vi "Autonomous Independent.vi"() -> ()   [LabVIEW 2015]
doc: "This VI is called when autonomous begins, and will automatically be terminated when autonomous ends. You can carry out timed or sensor driven robot movement independently without needing to return to the caller."
uses:
  navX-MXP Library/COMMON/TypeDefs/Data TypeDefs/navX Vector Data.ctl
  navX-MXP Library/COMMON/TypeDefs/Data TypeDefs/navX YPRH Data.ctl
  navX-MXP Library/COMMON/TypeDefs/Data TypeDefs/navX Quaternion Data.ctl
  Robot Global Data.vi
  navX-MXP Library/navX-MXP IMU.lvlib
  <vilib>/addons/control/pid/NI_PID_pid.lvlib
  <vilib>/addons/control/pid/pid.llb/PID (DBL).vi
panel:
  in  "PID gains":T1={"proportional gain (Kc)"=1.0, "integral time (Ti, min)"=0.01, "derivative time (Td, min)"=0.0} {"derivative time (Td, min)" format="%.3f"; "integral time (Ti, min)" format="%.3f"; "proportional gain (Kc)" format="%.3f"}
  in  "Drive Speed":dbl
  out "Quaternion":T2
  out "YPRH":T3
  out "Raw Magnetometer":T4
  out "Raw Gyro":T4
  out "Raw Acceleration":T4
  out "Fused Heading":dbl
  # "Be sure to right-click and choose Data Operations>>Make Current Value default if you want to save the array values with the VI"
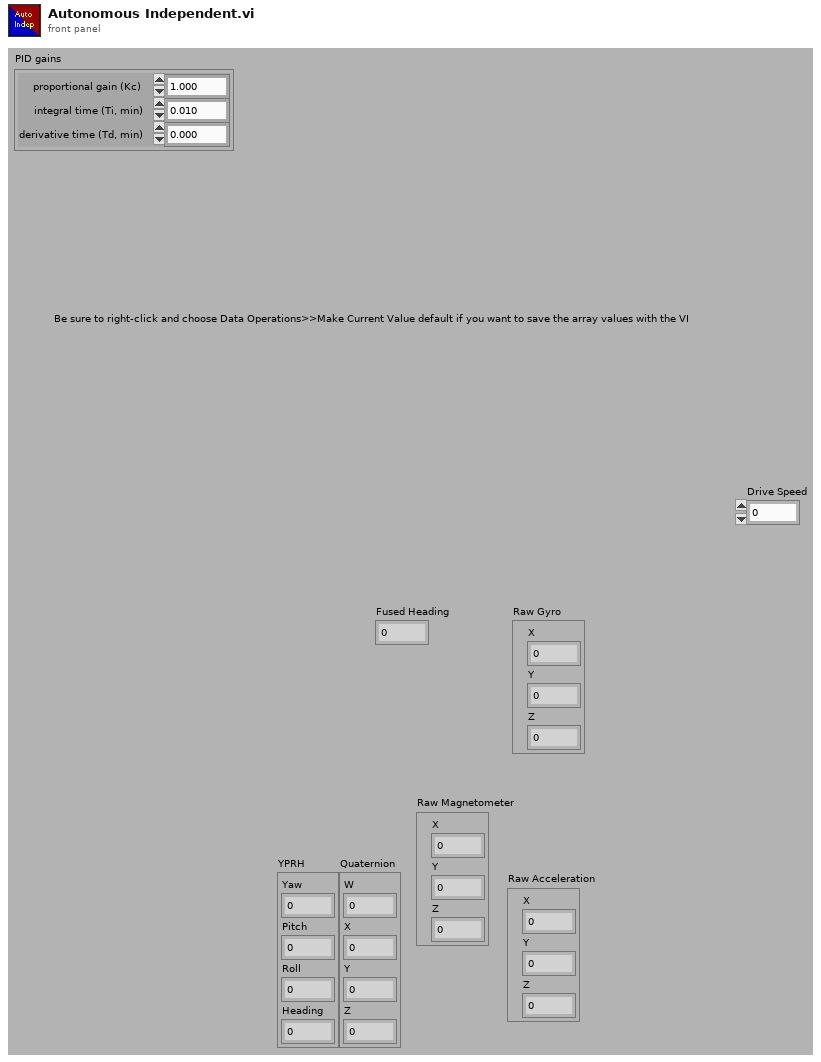
[diagram p1: front panel]
types:
  T1 = cluster{"proportional gain (Kc)":dbl, "integral time (Ti, min)":dbl, "derivative time (Td, min)":dbl}
  T2 = typedef "navX-MXP IMU.lvlib/navX Quaternion Data.ctl" = cluster{"W":dbl, "X":dbl, "Y":dbl, "Z":dbl}
  T3 = typedef "navX-MXP IMU.lvlib/navX YPRH Data.ctl" = cluster{"Yaw":dbl, "Pitch":dbl, "Roll":dbl, "Heading":dbl}
  T4 = typedef "navX-MXP IMU.lvlib/navX Vector Data.ctl" = cluster{"X":dbl, "Y":dbl, "Z":dbl}
  T5 = typedef "navX-MXP IMU.lvlib/navX Device TypeDef.ctl" = cluster{"navX Interface Protocol":T6, "navX Interface Protocol TypeDefs":cluster{"SPIDevRef":T7, "I2CDevRef":T9}, "navX System Information":cluster{"Board Information":T11, "Status":T14, "Offsets":T18, "LastSampleTimestamp":dbl, "LastSampleValid":bool}, "navX Common Information":cluster{"Update Rate (4Hz-60Hz)":T19, "refnum name":string, "error":errorcluster, "LastSampleFPGATimestamp":dbl}}
  T6 = typedef "navX-MXP IMU.lvlib/navX Interface Protocol.ctl" = enum16{"SPI", "I2C", "SERIAL"}
  T7 = typedef "WPI_SPIDevRef.ctl" = cluster{"DevStatus":errorcluster, "Handle":i32, "SPI Bus":T8}
  T8 = typedef "spi_bus.ctl" = enum16{"SPI On-Board, CS0", "SPI On-Board, CS1", "SPI On-Board, CS2", "SPI On-Board, CS3", "SPI MXP", "Invalid"}
  T9 = typedef "WPI_I2CDevRef.ctl" = cluster{"DevStatus":errorcluster, "Device Address":u8, "Handle":i32, "I2C Bus":T10}
  T10 = typedef "i2c_bus.ctl" = enum16{"I2C On-Board", "I2C MXP", "Invalid"}
  T11 = typedef "navX-MXP IMU.lvlib/navX Board Information.ctl" = cluster{"WhoAmI (50 | 0x32)":u8, "Board Revision":u8, "Firmware Major Version":u8, "Firmware Minor Version":u8, "NAVX_BOARD_CAPABILITY":T12, "NAVX_BOARD_YAW_AXIS":T13}
  T12 = typedef "navX-MXP IMU.lvlib/navX NAVX_BOARD_CAPABILITY.ctl" = cluster{"OMNIMOUNT":bool, "YAW_RESET":bool, "VEL_AND_DISP":bool}
  T13 = typedef "navX-MXP IMU.lvlib/navX NAVX_BOARD_YAW_AXIS.ctl" = cluster{"BOARD_YAW_AXIS_UP":bool, "BOARD_YAW_AXIS":u8}
  T14 = typedef "navX-MXP IMU.lvlib/navX Status Data.ctl" = cluster{"Update Rate Hz":u8, "Accelerometer Full-Scale Range":u8, "Gyro Full-Scale Range":u16, "NAVX_OP_STATUS":T15, "NAVX_CAL_STATUS":T16, "NAVX_SELFTEST_STATUS":u8, "NAVX_SENSOR_STATUS":T17}
  T15 = typedef "navX-MXP IMU.lvlib/navX NAVX_OP_STATUS.ctl" = u8
  T16 = typedef "navX-MXP IMU.lvlib/navX NAVX_CAL_STATUS.ctl" = u8
  T17 = typedef "navX-MXP IMU.lvlib/navX NAVX_SENSOR_STATUS.ctl" = cluster{"MOVING":bool, "YAW_STABLE":bool, "MAG_DISTURBANCE":bool, "ALTITUDE_VALID":bool, "SEALEVEL_PRESS_SET":bool, "FUSED_HEADING_VALID":bool}
  T18 = typedef "navX-MXP IMU.lvlib/navX Offsets Data.ctl" = cluster{"Yaw":dbl, "Quat W":dbl, "Quat X":dbl, "Quat Y":dbl, "Quat Z":dbl}
  T19 = typedef "navX-MXP IMU.lvlib/navX Update Rate.ctl" = u8
  T20 = typedef "WPI_MotorControlDeviceRef.ctl" = cluster{"DeviceStatus":errorcluster, "Type":T21, "PWM":cluster{"PWM Channel":T22, "DeadBand":T23}, "CAN":cluster{"Device Number":u8, "Control Mode":T24, "Semaphore":T25, "Max Vout":dbl, "TalonSRX Control Mode":T26}, "Invert":bool}
  T21 = typedef "WPI_MotorControlType.ctl" = enum16{"PWM", "CAN", "CANTalonSRX"}
  T22 = typedef "FPGA_DIOPWMChannel.ctl" = enum8{"PWM 0", "PWM 1", "PWM 2", "PWM 3", "PWM 4", "PWM 5", "PWM 6", "PWM 7", "PWM 8", "PWM 9", "PWM MXP 0", "PWM MXP 1", "PWM MXP 2", "PWM MXP 3", "PWM MXP 4", "PWM MXP 5", "PWM MXP 6", "PWM MXP 7", "PWM MXP 8", "PWM MXP 9", "Invalid"}
  T23 = typedef "WPI_PWMDeadband.ctl" = cluster{"Name":string, "maxPositivePwm":i32, "minPositivePwm":i32, "centerPwm":i32, "maxNegativePwm":i32, "minNegativePwm":i32, "angularRange":u16}
  T24 = typedef "WPI_CANJaguar_ControlMode.ctl" = enum8{"Percent VBus", "Current", "Speed", "Position", "Voltage"}
  T25 = typedef "Semaphore RefNum" = refnum<k1>
  T26 = typedef "WPI_CANTalonSRX_APIControlMode.ctl" = enum8{"Percent VBus", "Speed", "Position", "Slave", "Unchanged / Invalid", "Voltage Compensation", "Current", "Motion Profile"}
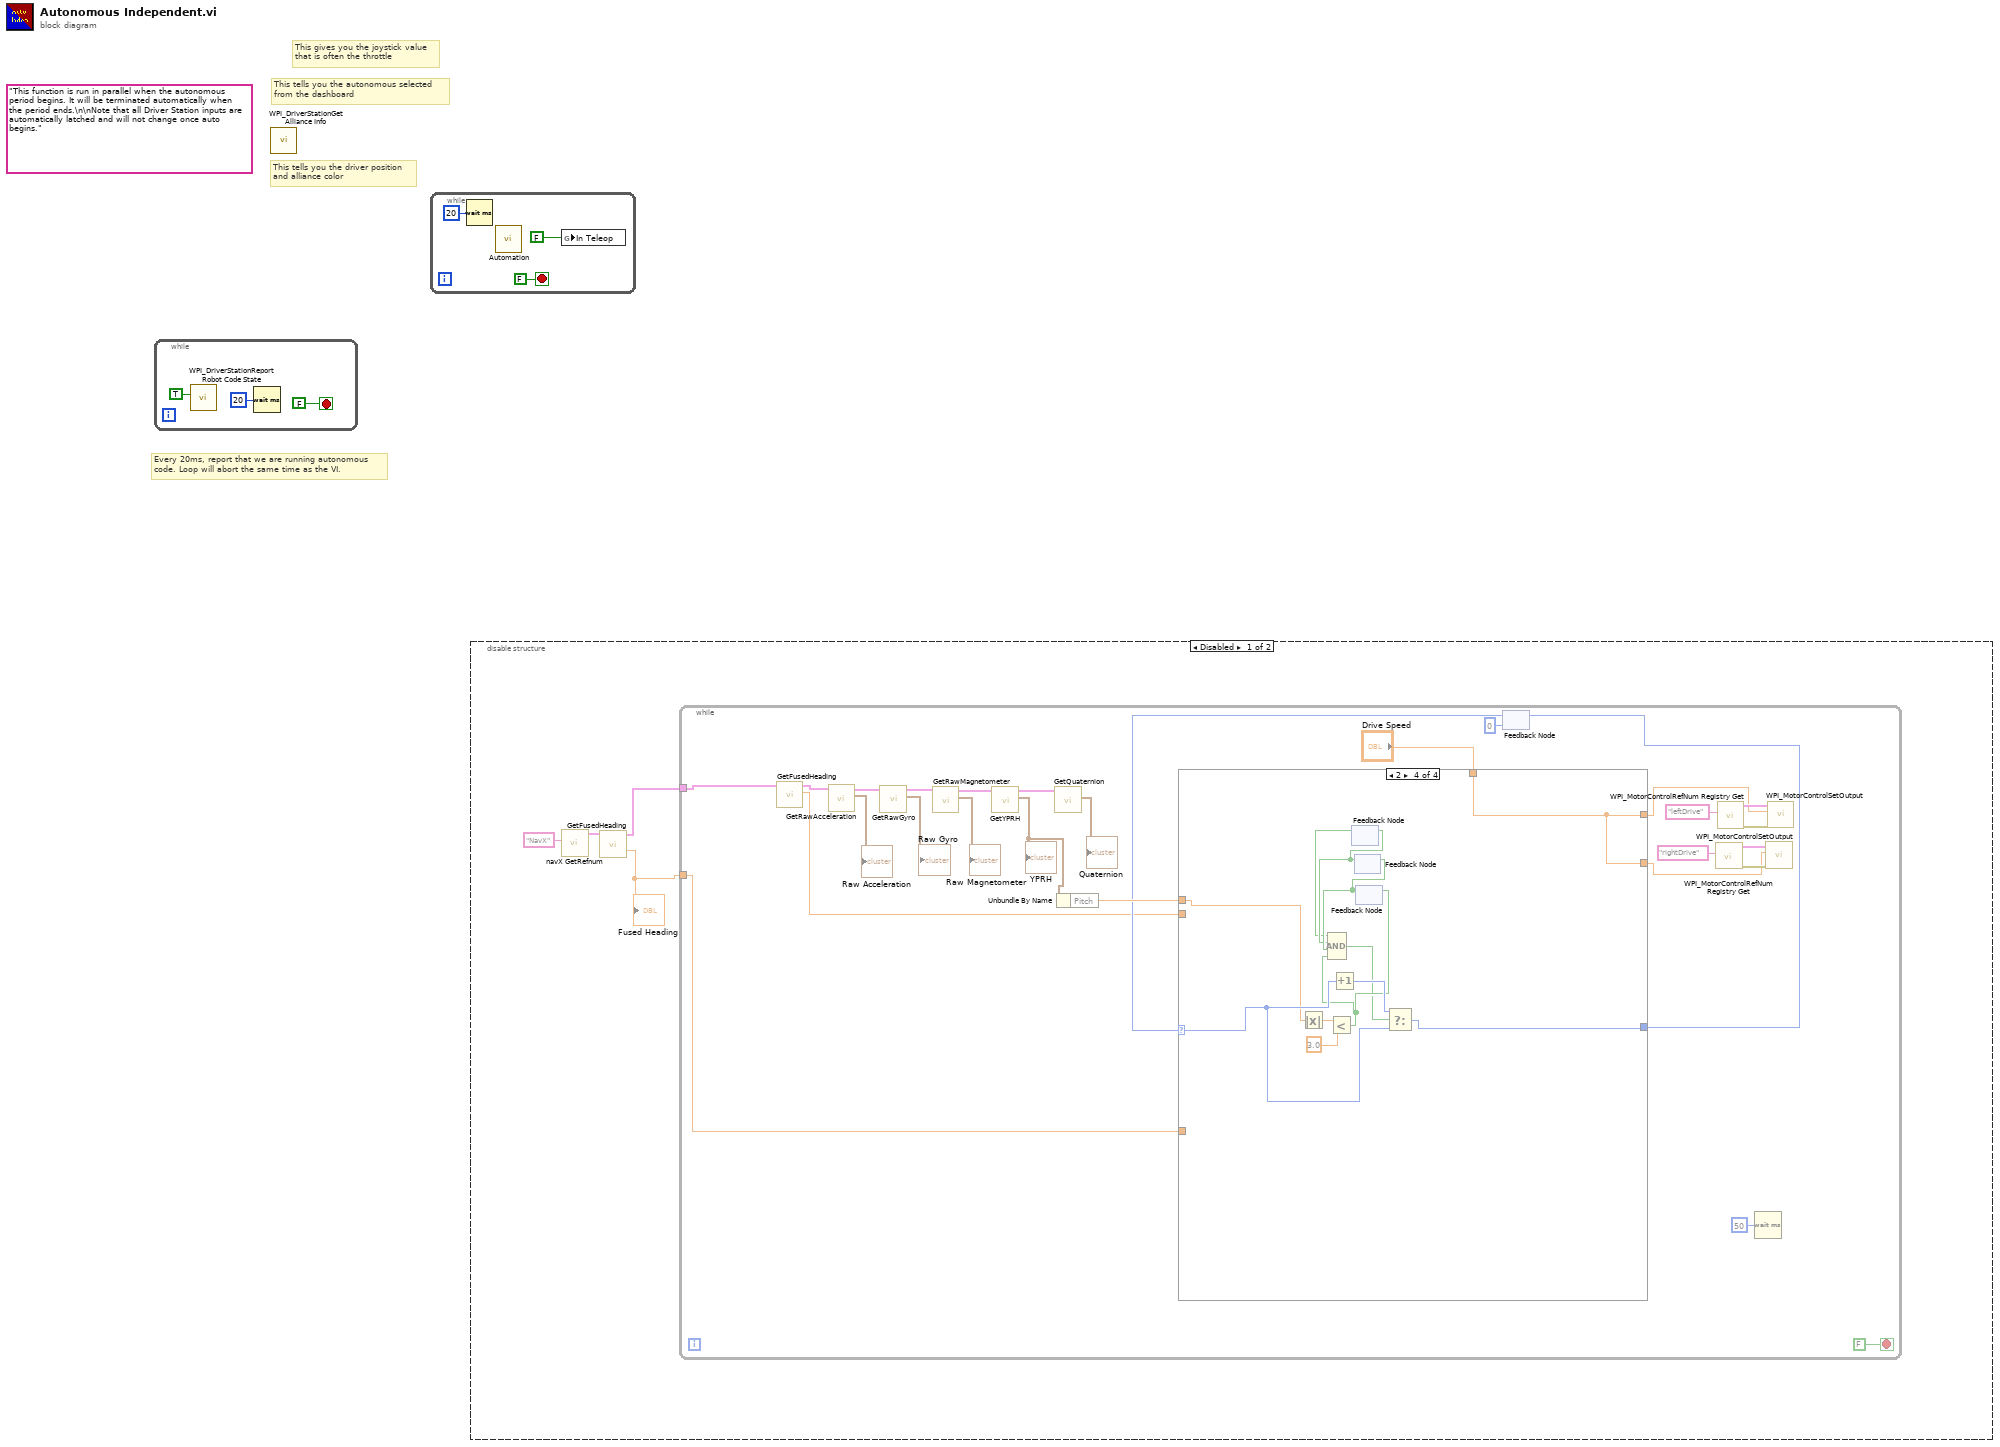
[diagram p0: block diagram]
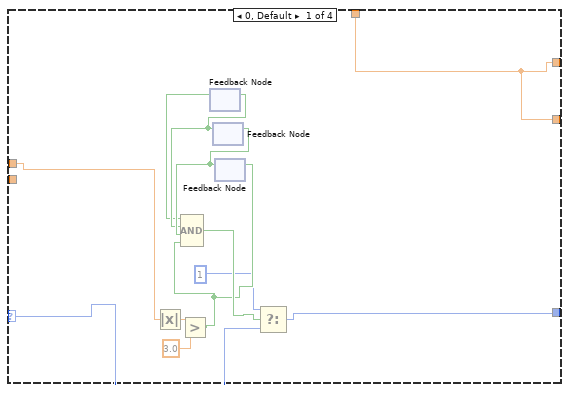
[diagram p2: hidden frame]
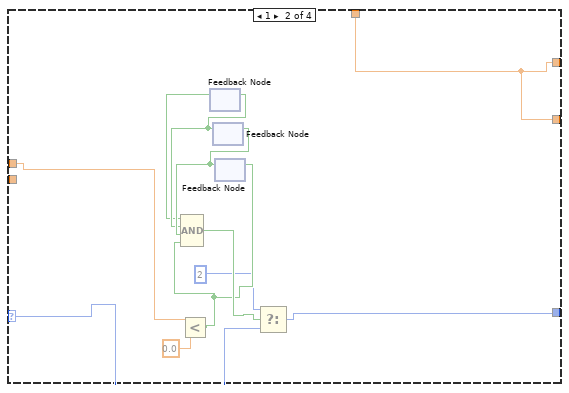
[diagram p3: hidden frame]
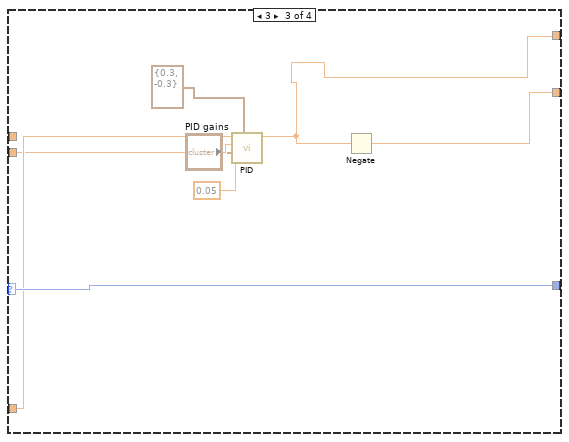
[diagram p4: hidden frame]
diagram:
  (unwired) "This function is run in parallel when the autonomous period begins. It will be terminated automatically when the period ends.\n\nNote that all Driver Station inputs are automatically latched and will not change once auto begins."
  # "This tells you the autonomous selected\nfrom the dashboard"
  # "Every 20ms, report that we are running autonomous\ncode. Loop will abort the same time as the VI."
  # "This gives you the joystick value\nthat is often the throttle"
  # "This tells you the driver position\nand alliance color"
  n1 = while {
    stop <- FALSE stop-if-true
    n2 = call <vilib>:"WPI_DriverStationReport Robot Code State.vi"("Autonomous"=TRUE) -> ()  [unwired: 10 in, 1 out]
    n3 = Wait (ms)(milliseconds to wait=u32 20) -> ()  [unwired: 1 out]
  }
  n4 = call <vilib>:"WPI_DriverStationGet Alliance Info.vi"() -> ()  [unwired: 12 out]
  n5 = while {
    stop <- FALSE stop-if-true
    n6 = Wait (ms)(milliseconds to wait=u32 20) -> ()  [unwired: 1 out]
    n7 = call "Automation.vi"() -> ()  [unwired: 12 in]
    n8 = global write "Robot Global Data.vi" "In Teleop"(FALSE ("Overide Drives")) -> ()
  }
  n9 = disable-structure shown="Disabled" {
    frame Disabled {
      n10 = call "navX GetRefnum.vi"("refnum name"="NavX") -> ("navX Device TypeDef"=w9:T5)  [unwired: 9 in, 1 out]
      n11 = call "GetFusedHeading.vi"("navX Device TypeDef"=w9) -> ("Fused Heading"=w8:dbl, "navX Device TypeDef"=w7:T5)  [unwired: 8 in, 1 out]
      "Fused Heading" <- w8
      n12 = while {
        tunnel: w8 -> [w12]
        tunnel: w7 -> [w13]
        stop <- FALSE stop-if-true
        n13 = call "GetFusedHeading.vi"("navX Device TypeDef"=w13) -> ("Fused Heading"=w11:dbl, "navX Device TypeDef"=w14:T5)  [unwired: 8 in, 1 out]
        n14 = call "GetRawAcceleration.vi"("navX Device TypeDef"=w14) -> ("Raw Acceleration"=→"Raw Acceleration":T4, "navX Device TypeDef"=w30:T5)  [unwired: 8 in, 1 out]
        n15 = call "GetRawGyro.vi"("navX Device TypeDef"=w30) -> ("Raw Gyro"=→"Raw Gyro":T4, "navX Device TypeDef"=w28:T5)  [unwired: 8 in, 1 out]
        n16 = call "GetRawMagnetometer.vi"("navX Device TypeDef"=w28) -> ("Raw Magnetometer"=→"Raw Magnetometer":T4, "navX Device TypeDef"=w26:T5)  [unwired: 8 in, 1 out]
        n17 = call "GetYPRH.vi"("navX Device TypeDef"=w26) -> ("YPRH"=w23:T3, "navX Device TypeDef"=w25:T5)  [unwired: 8 in, 1 out]
        "YPRH" <- w23
        n18 = call "GetQuaternion.vi"("navX Device TypeDef"=w25) -> ("Quaternion"=→"Quaternion":T2)  [unwired: 8 in, 2 out]
        n19 = Unbundle By Name(w23) -> ("Pitch"=w22:dbl)
        n20 = feedback #1(0) -> (w17:i32)
        n21 = case shown="2" w17 {
          selector: w17 -> [w49 w61 w69 w78]
          tunnel: w22 -> [w50 w51 _ w76]
          tunnel: "Drive Speed" -> [w40 w53 _ w70]
          tunnel: [w40 w53 w62 w70] -> w19
          tunnel: [w40 w53 w63 w70] -> w20
          tunnel: [w48 w60 w69 w77] -> w18
          tunnel: w12 -> [_ _ w68 _]
          tunnel: w11 -> [_ _ w67 _]
          frame 0, Default {
            n22 = Absolute Value(x=w50) -> (abs(x)=w47:dbl)
            n23 = Greater?(x=w47, y=3.0) -> (0:w41:bool)
            n24 = feedback #2() -> (w43:bool)  [unwired: 1 in]
            n25 = feedback #3() -> (w44:bool)  [unwired: 1 in]
            n26 = feedback-in #2(w44) -> ()
            n27 = feedback #4() -> (w45:bool)  [unwired: 1 in]
            n28 = Compound Arithmetic op=AND(w43, w44, w45, w41) -> (w42:bool)
            n29 = feedback-in #3(w45) -> ()
            n30 = feedback-in #4(w41) -> ()
            n31 = Select(t=1, s=w42, f=w49) -> (s? t:f=w48:i32)
          }
          frame 1 {
            n32 = Less?(x=w51, y=0.0) -> (x < y?=w54:bool)
            n33 = feedback #5() -> (w56:bool)  [unwired: 1 in]
            n34 = feedback #6() -> (w57:bool)  [unwired: 1 in]
            n35 = feedback-in #5(w57) -> ()
            n36 = feedback #7() -> (w58:bool)  [unwired: 1 in]
            n37 = Compound Arithmetic op=AND(w56, w57, w58, w54) -> (w55:bool)
            n38 = feedback-in #6(w58) -> ()
            n39 = feedback-in #7(w54) -> ()
            n40 = Select(t=2, s=w55, f=w61) -> (s? t:f=w60:i32)
          }
          frame 3 {
            n41 = call-poly <vilib>:"PID.vi"("output range"=cluster{"output high":dbl, "output low":dbl} {"output high"=0.3, "output low"=-0.3}, "dt (s)"=0.05, "PID gains"="PID gains", "process variable"=w67, "setpoint"=w68) -> ("output"=w62:dbl)  [unwired: 5 in, 1 out]
            n42 = Negate(x=w62) -> (-x=w63:dbl)
          }
          frame 2 {
            n43 = Absolute Value(x=w76) -> (abs(x)=w81:dbl)
            n44 = Less?(x=w81, y=3.0) -> (x < y?=w75:bool)
            n45 = Increment(x=w78) -> (x+1=w79:i32)
            n46 = feedback #8() -> (w72:bool)  [unwired: 1 in]
            n47 = feedback #9() -> (w73:bool)  [unwired: 1 in]
            n48 = feedback-in #8(w73) -> ()
            n49 = feedback-in #10(w75) -> ()
            n50 = feedback #10() -> (w74:bool)  [unwired: 1 in]
            n51 = Compound Arithmetic op=AND(w72, w73, w74, w75) -> (w71:bool)
            n52 = feedback-in #9(w74) -> ()
            n53 = Select(t=w79, s=w71, f=w78) -> (s? t:f=w77:i32)
          }
        }
        n54 = feedback-in #1(w18) -> ()
        n55 = call <vilib>:"WPI_MotorControlRefNum Registry Get.vi"("refnum name"="rightDrive") -> ("error out"=w32:errorcluster, "MotorControlDevRef"=w33:T20)  [unwired: 9 in]
        n56 = call <vilib>:"WPI_MotorControlRefNum Registry Get.vi"("refnum name"="leftDrive") -> ("error out"=w37:errorcluster, "MotorControlDevRef"=w36:T20)  [unwired: 9 in]
        n57 = Wait (ms)(milliseconds to wait=u32 50) -> ()  [unwired: 1 out]
        n58 = call <vilib>:"WPI_MotorControlSetOutput.vi"("error in (no error)"=w32, "Output"=w20, "MotorControlDevRef"=w33) -> ()  [unwired: 6 in, 3 out]
        n59 = call <vilib>:"WPI_MotorControlSetOutput.vi"("error in (no error)"=w37, "Output"=w19, "MotorControlDevRef"=w36) -> ()  [unwired: 6 in, 3 out]
      }
    }
    frame Enabled {
    }
  }
